vi "Task_initiation.vi"() -> (0 "task out\nlaser trigger":refnum<k21>, 1 "task out\nedge count":refnum<k21>, 2 "task out CC":refnum<k21>)   [LabVIEW 2016]
uses:
  <vilib>/DAQmx/write.llb/DAQmx Write (Analog DBL 1Chan 1Samp).vi
  <vilib>/DAQmx/create/channels.llb/DAQmx Create Channel (AO-Voltage-Basic).vi
  <vilib>/DAQmx/miscellaneous.llb/DAQmx Fill In Error Info.vi
  Utility/Global Constants.vi
  <vilib>/DAQmx/create/channels.llb/DAQmx Create Channel (CI-Count Edges).vi
  <resource>/objmgr/daqmx.rc
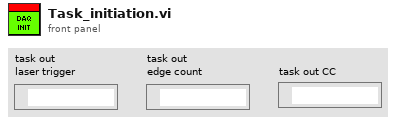
[diagram p1: front panel]
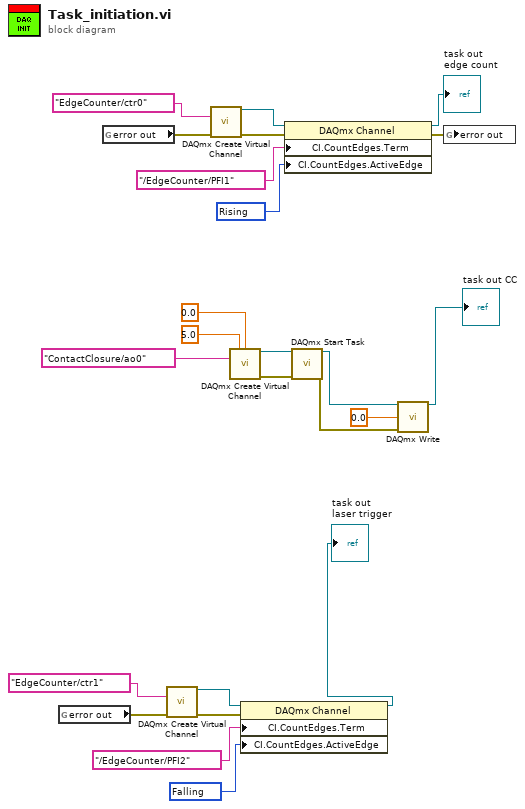
[diagram p0: block diagram]
diagram:
  w15 = 10171 items=["Rising"=10280, "Falling"=10171] ("Active Edge")
  w23 = 10280 items=["Rising"=10280, "Falling"=10171] ("Active Edge")
  n1 = global read "Global Constants.vi" "error out"() -> (w11:errorcluster)
  n2 = global read "Global Constants.vi" "error out"() -> (w19:errorcluster)
  n3 = call-poly <vilib>:"DAQmx Create Virtual Channel.vi"("counter"=tag "EdgeCounter/ctr1" ("Counter"), "error in"=w11) -> ("task out"=w13:refnum<k21>, "error out"=w12:errorcluster)  [unwired: 12 in]
  n4 = call-poly <vilib>:"DAQmx Create Virtual Channel.vi"("counter"=tag "EdgeCounter/ctr0" ("Counter"), "error in"=w19) -> ("task out"=w21:refnum<k21>, "error out"=w20:errorcluster)  [unwired: 12 in]
  n5 = call-poly <vilib>:"DAQmx Create Virtual Channel.vi"("maximum value"=5.0 ("Max Voltage"), "minimum value"=0.0 ("Min Voltage"), "physical channels"=tag "ContactClosure/ao0" ("Physical Channel(s)")) -> ("task out"=w6:refnum<k21>, "error out"=w5:errorcluster)  [unwired: 11 in]
  n6 = property class="DAQmx Channel"(reference=w13, error in=w12, "CI.CountEdges.Term"=tag "/EdgeCounter/PFI2" ("Input Terminal"), "CI.CountEdges.ActiveEdge"=w15) -> (reference out=→"task out\nlaser trigger":refnum<k21>)  [unwired: 1 out]
  n7 = property class="DAQmx Channel"(reference=w21, error in=w20, "CI.CountEdges.Term"=tag "/EdgeCounter/PFI1" ("Input Terminal"), "CI.CountEdges.ActiveEdge"=w23) -> (reference out=→"task out\nedge count":refnum<k21>, error out=w17:errorcluster)
  n8 = call <vilib>:"DAQmx Start Task.vi"("task/channels in"=w6, "error in"=w5) -> ("task out"=w4:refnum<k21>, "error out"=w3:errorcluster)  [unwired: 12 in]
  n9 = call-poly <vilib>:"DAQmx Write.vi"("task/channels in"=w4, "data"=0.0, "error in"=w3) -> ("task out"=→"task out CC":refnum<k21>)  [unwired: 10 in, 2 out]
  n10 = global write "Global Constants.vi" "error out"(w17) -> ()
